vi "(TestVI)HTTP Get File Download.vi"() -> ()   [LabVIEW 2020]
uses:
  <vilib>/httpClient/LabVIEWHTTPClient.lvlib
panel:
  out "길이":i32
  out "body":string caption="본문"
  out "headers":string caption="헤더"
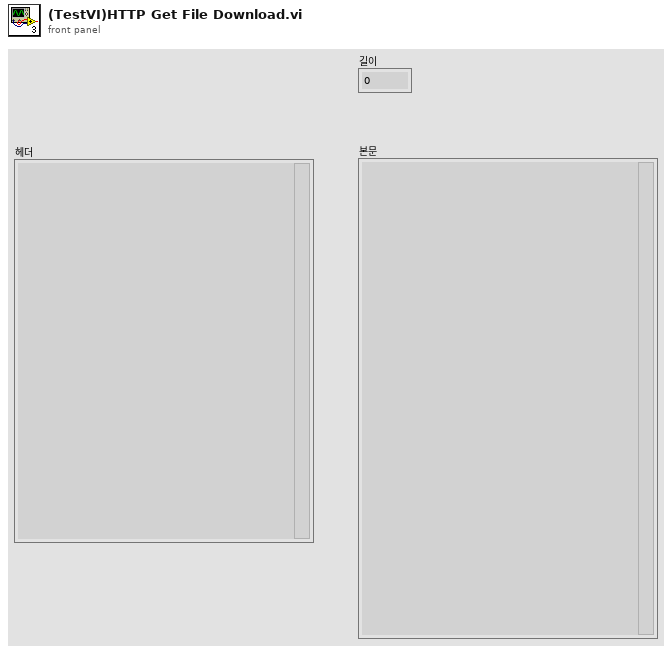
[diagram p1: front panel]
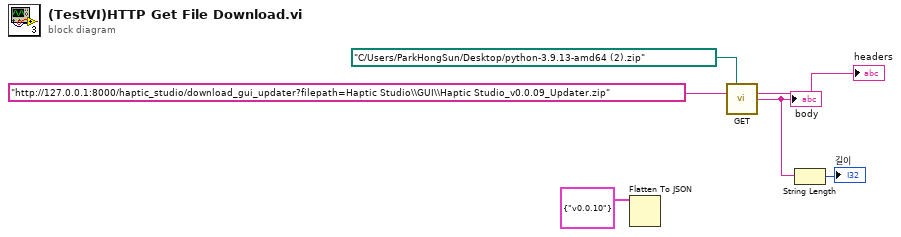
[diagram p0: block diagram]
diagram:
  n1 = Flatten To JSON(anything=cluster{"version":string} {"version"="v0.0.10"}) -> ()  [unwired: 2 in, 2 out]
  n2 = call <vilib>:"GET.vi"("output file"=path "C:/Users/ParkHongSun/Desktop/python-3.9.13-amd64 (2).zip", "url"="http://127.0.0.1:8000/haptic_studio/download_gui_updater?filepath=Haptic Studio\\GUI\\Haptic Studio_v0.0.09_Updater.zip") -> ("headers"=→"headers":string, "body"=w3:string)  [unwired: 10 in, 2 out]
  "body" <- w3
  n3 = String Length(string=w3) -> (length=→"길이":i32)
